vi "Save_SetParas.vi"(7 "cmd":T1, 8 "error in (no error)":errorcluster caption="에러 입력(에러 없음)", 9 "Data":string="First\nData\nString", 10 "Key":string="String1", 11 "Section":string="Conditions") -> (0 "error out":errorcluster caption="에러 출력", 3 "dataout":cluster{"DataOut":string, "exist":bool})   [LabVIEW 2019]
uses:
  cmd_setPara.ctl
  <vilib>/Utility/config.llb/Write Key (String).vi
  <vilib>/Utility/config.llb/Read Key (String).vi
  <vilib>/Utility/config.llb/NI_LVConfig.lvlib
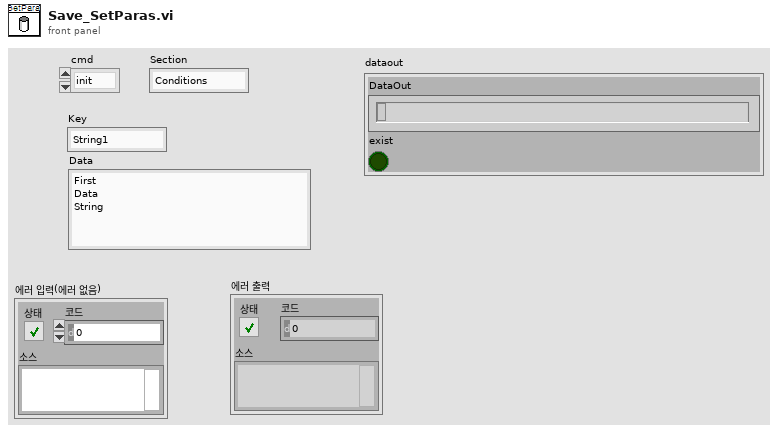
[diagram p1: front panel]
types:
  T1 = typedef "cmd_setPara.ctl" = enum16{"init", "write", "read", "default"}
  T2 = typedef "NI_LVConfig.lvlib/Config Data RefNum.ctl" = refnum<k1>
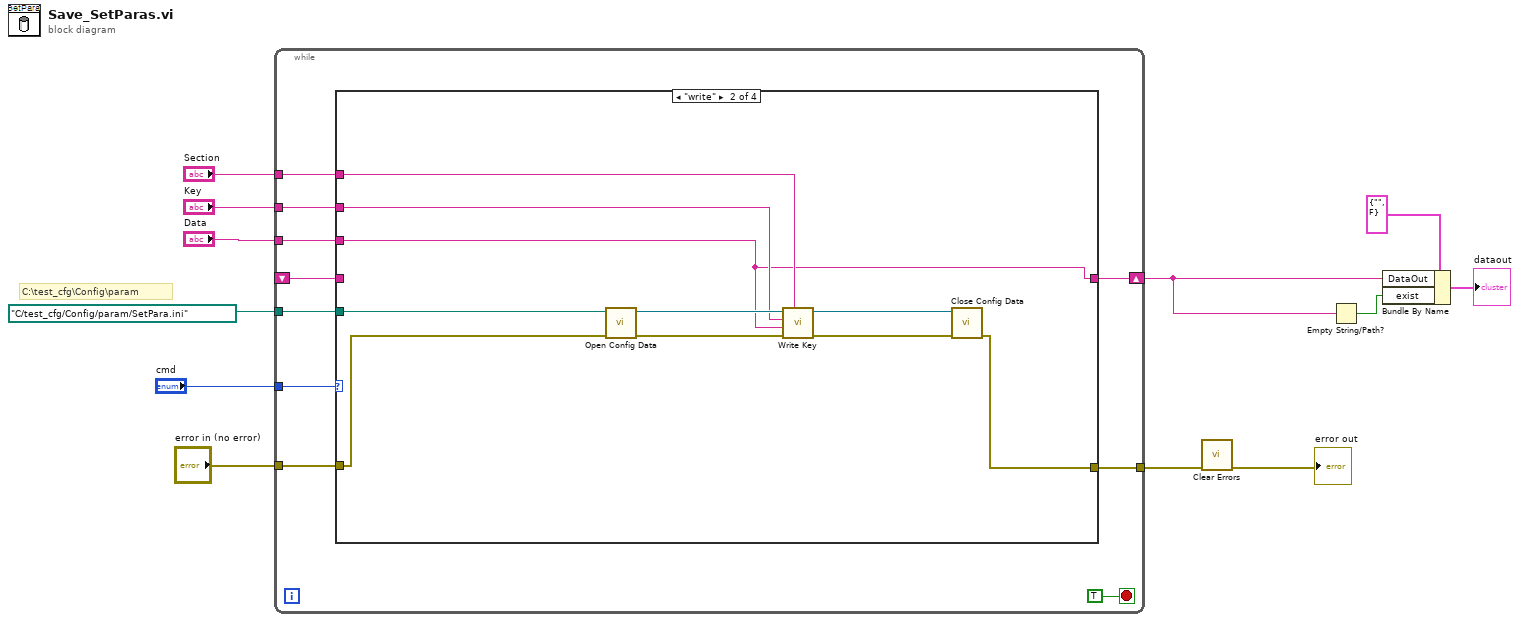
[diagram p0: block diagram]
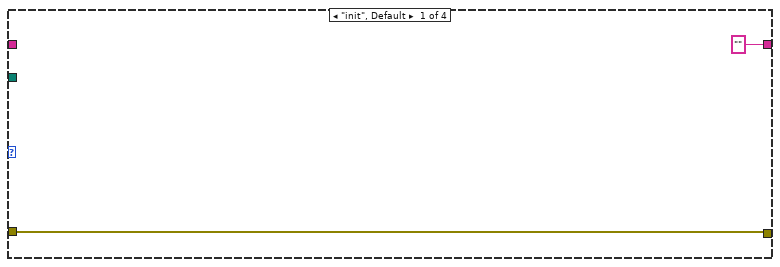
[diagram p2: hidden frame]
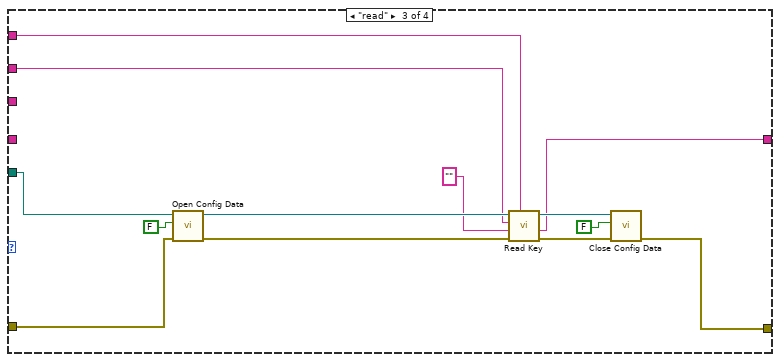
[diagram p3: hidden frame]
diagram:
  # "C:\\test_cfg\\Config\\param"
  n1 = while {
    tunnel: "cmd" -> [w21]
    tunnel: "Section" -> [w20]
    tunnel: "Key" -> [w19]
    tunnel: "Data" -> [w18]
    tunnel: path "C:/test_cfg/Config/param/SetPara.ini" ("configuration file path") -> [w17]
    shift-right: [w16] -> w4
    shift-left: _ -> [w15]
    tunnel: "error in (no error)" -> [w14]
    tunnel: [w13] -> w6
    stop <- TRUE stop-if-true
    n2 = case shown="\"write\"" w21 {
      tunnel: w20 -> [_ w30 w40 _]
      tunnel: w19 -> [_ w29 w39 _]
      tunnel: w18 -> [_ w27 _ _]
      tunnel: w17 -> [_ w28 w41 _]
      tunnel: ["" ("value") w27 w38 w49] -> w16
      tunnel: w15 -> [_ _ _ w49]
      tunnel: w14 -> [w23 w26 w37 w48]
      tunnel: [w23 w25 w36 w48] -> w13
      frame "init", Default {
      }
      frame "write" {
        n3 = call <vilib>:"Open Config Data.vi"("error in (no error)"=w26, "configuration file path"=w28) -> ("error out"=w32:errorcluster, "refnum"=w31:T2)  [unwired: 1 in, 7 out]
        n4 = call-poly <vilib>:"Write Key.vi"("section"=w30, "error in (no error)"=w32, "value"=w27, "key"=w29, "refnum"=w31) -> ("error out"=w34:errorcluster, "refnum out"=w33:T2)  [unwired: 1 in, 4 out]
        n5 = call <vilib>:"Close Config Data.vi"("error in (no error)"=w34, "refnum"=w33) -> ("error out"=w25:errorcluster)  [unwired: 1 in, 8 out]
      }
      frame "read" {
        n6 = call <vilib>:"Open Config Data.vi"("error in (no error)"=w37, "create file if necessary (T)"=FALSE ("create file if necessary? (T)"), "configuration file path"=w41) -> ("error out"=w47:errorcluster, "refnum"=w46:T2)  [unwired: 6 in, 1 out]
        n7 = call-poly <vilib>:"Read Key.vi"("section"=w40, "error in (no error)"=w47, "default value"="", "key"=w39, "refnum"=w46) -> ("error out"=w44:errorcluster, "value"=w38:string, "refnum out"=w45:T2)  [unwired: 3 in, 1 out]
        n8 = call <vilib>:"Close Config Data.vi"("error in (no error)"=w44, "write file if changed (T)"=FALSE ("write configuration file? (T)"), "refnum"=w45) -> ("error out"=w36:errorcluster)  [unwired: 8 out]
      }
      frame "default" {
      }
    }
  }
  n9 = call <vilib>:"Clear Errors.vi"("error in (no error)"=w6) -> ("error out"=→"error out":errorcluster)  [unwired: 5 in, 1 out]
  n10 = Empty String/Path?(string/path=w4) -> (empty?=w3:bool)
  n11 = Bundle By Name(cluster=cluster{"DataOut":string, "exist":bool} {"DataOut"="", "exist"=FALSE} ("dataout"), "DataOut"=w4, "exist"=w3) -> (→"dataout":cluster{"DataOut":string, "exist":bool})
